vi "mhk_velmex_ice3.vi"() -> ()   [LabVIEW 2010]
panel:
  in  "VISA resource name":refnum<visa-resource-name>
  out "Command String":string
  in  "Number of Steps":u32(knob)=1 min=1 max=100000 step=1 scale=1.0..100000.0
  in  "Direction":bool
  in  "Motor Speed\n(Steps/sec)":i32(knob)=2000 min=2000 max=8000 scale=2000.0..8000.0
  in  "Motor Number":dbl=1.0 min=1.0 max=4.0 step=1.0
  # "Negative"
  # "Positive"
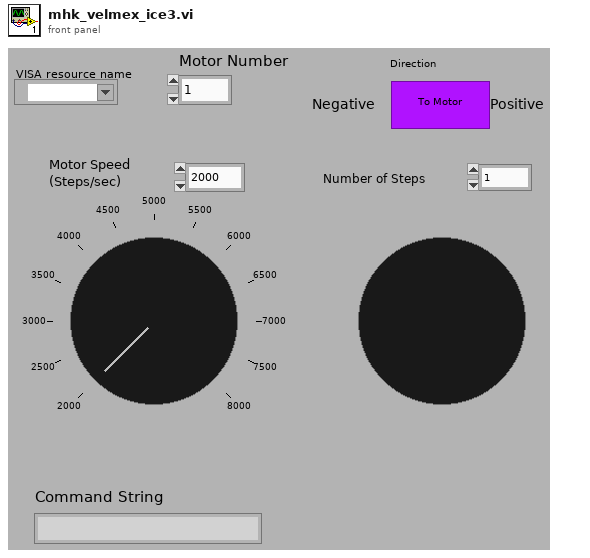
[diagram p1: front panel]
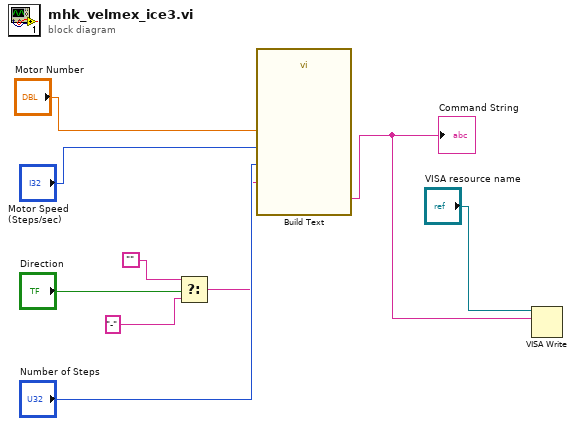
[diagram p0: block diagram]
diagram:
  n1 = Select(t="", s="Direction", f="-") -> (s? t:f=w2:string)
  n2 = call "Build Text"("Number of Steps"="Number of Steps", "Motor Number"="Motor Number", "Motor Speed"="Motor Speed\n(Steps/sec)", "Direction"=w2) -> ("Result"=w1:string)  [unwired: 10 in, 1 out]
  "Command String" <- w1
  n3 = VISA Write(VISA resource name="VISA resource name", write buffer=w1) -> ()  [unwired: 1 in, 3 out]
